vi "Init Msg.vi"(6 "Teller":refnum<class "Teller.lvclass">, 10 "Safe":bool=TRUE) -> (2 "Msg":refnum<class "Msg.lvclass">)   [LabVIEW 2020, in "jettl.lvlib" / "Stop jettl Msg.lvlib" / "Stop.lvlib"]
uses:
  Stop.lvlib
  Teller/Teller.lvclass
  Msg/Msg.lvclass
  Stop Msg/Stop Msg.lvlib
  Stop Msg Input/Stop Msg Input.lvlib
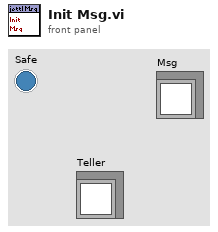
[diagram p1: front panel]
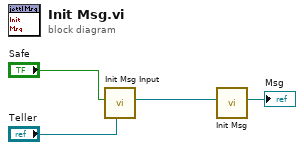
[diagram p0: block diagram]
diagram:
  n1 = call "Init Msg Input.vi"("Teller"="Teller", "Safe"="Safe") -> ("Msg Input"=w2:refnum<class "Msg Input.lvclass">)  [unwired: 9 in]
  n2 = call "Init Msg.vi"("Msg Input"=w2) -> ("Msg"=→"Msg":refnum<class "Msg.lvclass">)  [unwired: 10 in]
